vi "Pre Launch Init.vi"(11 "GenericController in":refnum<class "GenericController.lvclass">) -> (0 "error out":errorcluster, 3 "GenericController out":refnum<class "GenericController.lvclass">)   [LabVIEW 2020, in "GenericController.lvlib" / "GenericController.lvclass"]
doc: "(<B>Filename</B>: Actor Framework.lvlib:Actor.lvclass:Pre Launch Init.vi)\n\nDefines behavior that occurs after the Launch Nested Actor method is invoked but before the actor's Actor Core method begins running.\n\nBy default, this method does nothing. A descendant class may override it to define behavior."
uses:
  GenericController.lvclass
  <vilib>/ActorFramework/Actor/Actor.lvclass
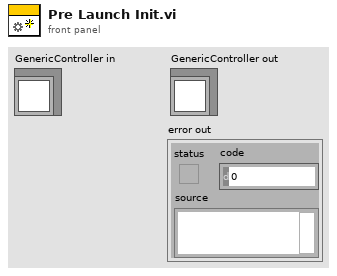
[diagram p1: front panel]
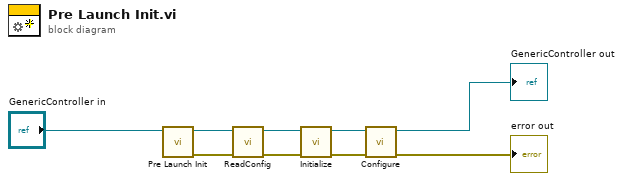
[diagram p0: block diagram]
diagram:
  n1 = call-parent "Pre Launch Init.vi"("Actor in"="GenericController in") -> ("error out"=w1:errorcluster, "Actor out"=w2:refnum<class "GenericController.lvclass">)  [unwired: 9 in]
  n2 = call-dynamic "ReadConfig.vi"("error in (no error)"=w1, "GRMActor in"=w2) -> ("error out"=w6:errorcluster, "GRMActor out"=w5:refnum<class "GenericController.lvclass">)  [unwired: 8 in]
  n3 = call-dynamic "Initialize.vi"("error in (no error)"=w6, "GRMActor in"=w5) -> ("error out"=w4:errorcluster, "GRMActor out"=w3:refnum<class "GenericController.lvclass">)  [unwired: 8 in]
  n4 = call-dynamic "Configure.vi"("error in (no error)"=w4, "GRMActor in"=w3) -> ("error out"=→"error out":errorcluster, "GRMActor out"=→"GenericController out":refnum<class "GenericController.lvclass">)  [unwired: 8 in]
